vi "SetSTimer.vi"(8 "error in (no error)":errorcluster) -> (0 "error out":errorcluster)   [LabVIEW 2015, in "ESLSCDLL.lvlib"]
uses:
  ESLSCDLL.lvlib
  Globals.vi
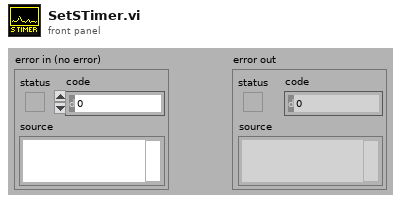
[diagram p1: front panel]
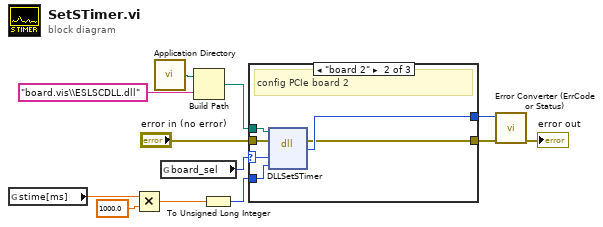
[diagram p0: block diagram]
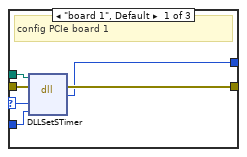
[diagram p2: hidden frame]
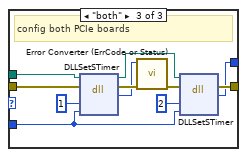
[diagram p3: hidden frame]
diagram:
  n1 = global read "Globals.vi" "stime[ms]"() -> (w5:dbl)
  n2 = Multiply(x=w5, y=1000.0) -> (x*y=w6:dbl)
  n3 = call <vilib>:"Application Directory.vi"() -> ("Application Directory"=w3:path)
  n4 = global read "Globals.vi" "board_sel"() -> (w8:enum32{"0", "board 1", "board 2", "both"})
  n5 = Build Path(base path=w3, name or relative path="board.vis\\ESLSCDLL.dll") -> (appended path=w1:path)
  n6 = To Unsigned Long Integer(number=w6) -> (unsigned 32bit integer=w4:u32)
  n7 = case shown="\"board 2\"" w8 {
    selector: w8 -> [w18 w24 _]
    tunnel: w4 -> [w17 w23 w33]
    tunnel: "error in (no error)" -> [w16 w20 w30]
    tunnel: [w15 w21 w28] -> w10
    tunnel: [w14 w22 w27] -> w9
    tunnel: w1 -> [w13 w19 w26]
    frame "board 1", Default {
      # "config PCIe board 1"
      n8 = dll-call lib="C:/ENTW/PCIE/LV64/board.vis/ESLSCDLL.dll" fn="DLLSetSTimer" ("lwlscdll.dll:DLLSetTemp")(path in=w13, error in=w16, "drv"=w18, "stime_in_microseconds"=w17) -> (error out=w15:errorcluster, "es_status_codes"=w14:i32)  [unwired: 3 in, 1 out]
    }
    frame "board 2" {
      # "config PCIe board 2"
      n9 = dll-call lib="C:/ENTW/PCIE/LV64/board.vis/ESLSCDLL.dll" fn="DLLSetSTimer" ("lwlscdll.dll:DLLSetTemp")(path in=w19, error in=w20, "drv"=w24, "stime_in_microseconds"=w23) -> (error out=w21:errorcluster, "es_status_codes"=w22:i32)  [unwired: 3 in, 1 out]
    }
    frame "both" {
      # "config both PCIe boards"
      n10 = dll-call lib="C:/ENTW/PCIE/LV64/board.vis/ESLSCDLL.dll" fn="DLLSetSTimer" ("lwlscdll.dll:DLLSetTemp")(path in=w26, error in=w30, "drv"=u32 1, "stime_in_microseconds"=w33) -> (path out=w25:path, error out=w32:errorcluster, "es_status_codes"=w31:i32)  [unwired: 3 in]
      n11 = call "Error Converter (ErrCode or Status).vi"("error in (no error)"=w32, "error code"=w31) -> ("error out"=w29:errorcluster)  [unwired: 9 in]
      n12 = dll-call lib="C:/ENTW/PCIE/LV64/board.vis/ESLSCDLL.dll" fn="DLLSetSTimer" ("lwlscdll.dll:DLLSetTemp")(path in=w25, error in=w29, "drv"=u32 2, "stime_in_microseconds"=w33) -> (error out=w28:errorcluster, "es_status_codes"=w27:i32)  [unwired: 3 in, 1 out]
    }
  }
  n13 = call "Error Converter (ErrCode or Status).vi"("error in (no error)"=w10, "error code"=w9) -> ("error out"=→"error out":errorcluster)  [unwired: 9 in]
